vi "00_FRA_sensors_main.vi"() -> ()   [LabVIEW 2013]
uses:
  subVIs/Sensor_power_ctrl.ctl
  subVIs/Unit_select_s_m.ctl
  subVIs/UDP_read_datagram.ctl
  subVIs/UI_states.ctl
  subVIs/Global Status bar event.vi
  subVIs/loop error, restart vi_err_cluster.vi
  subVIs/loop error, restart vi.vi
  <vilib>/Utility/file.llb/Read From Spreadsheet File (string).vi
panel:
  out "Status Bar VI":string
  out "Status":string="Ready!"
  in  "Tab Control":enum32{"Settings", "Measurement", "Log", "."}(tab)
  in  "Unit select single/mult 2":T1 caption="Unit selection \nsingle/multiple"
  in  "UseAMO":bool caption="Use Amonia Sensor"
  in  "MODECN":u8 format="%08b"
  in  "REFCN":u8 format="%08b"
  in  "TIACN":u8=18 format="%05b"
  in  "Conf.set":u8=6 caption="Configuration set (Electrochemical) (0-15)" max=15 step=1
  out "ACK'd_clients":u8[](array[numeric])
  out "Number of clients":i32
  out "Export Folder Path":path
  in  "Unit selection":u8=255
  in  "Reset Unit":bool
  in  "Trigger ON":bool
  in  "Trigger OFF":bool
  in  "Period (s)":sgl=1.0 min=0.1 max=25 step=0.1
  in  "Unit selection multiple":string[][](table)
  out "Unit display A":dbl[][](graph)=[[528.1875, 527.4375, 528.1875, 527.25, 525.75, 520.125, 579.0, 800.8125, 526.6875, 524.25, 525.0, 525.1875]]
  in  "unit to show A":u8=13
  out "Unit display B":dbl[][](graph)=[[543.375, 541.5, 544.875, 5008.6875, 535.6875, 535.3125, 535.875, 537.5625, 538.3125, 0.5625, 571.6875, 538.3125]]
  in  "unit to show C":u8=11
  in  "unit to show D":u8=12
  out "Unit display D":dbl[][](graph)=[[-0.01530459835686071, -0.000554118739038989, 0.03629888532152492, 0.0025318779311733763, 0.030571059615454033, 0.00759975996654827, 0.0011509882323559317, 0.003101779382480796, 0.003088657192881872, -0.0032983569178113292, -0.0038528679526479426, 1.0]]
  out "Unit display C":dbl[][](graph)=[[-0.01530459835686071, -0.000554118739038989, 0.03629888532152492, 0.0025318779311733763, 0.030571059615454033, 0.00759975996654827, 0.0011509882323559317, 0.003101779382480796, 0.003088657192881872, -0.0032983569178113292, -0.0038528679526479426, 1.0]]
  in  "unit to show B":u8=14
  out "Dead Units":u8[](array[numeric])
  out "Logged status messages":string[][](table)
  out "Unit selection merged":u8[][](array[numeric])
  in  "update_legends":bool
  out "Alive Units":u8[](array[numeric])
  out "Answer_received_from":u8[](array[numeric])
  in  "Unit port":u16=65500
  out "Data file ref":refnum<file>
  in  "Sensor power control":T2={"Power A1.0"=TRUE, "Power A1.1"=TRUE, "Power A1.2"=TRUE, "Power A1.3"=TRUE, "Power A2.0"=TRUE, "Power A2.1"=TRUE, "Power A2.2"=TRUE, "Power A2.3"=TRUE, "Power A3.1"=TRUE, "Power A3.2"=TRUE}
  in  "Power all sensors ON/OFF":bool
  out "ACK'd_clients addr":u32[](array[numeric]) format="%x"
  out "address":u32 format="%08x"
  out "data received":string
  out "Datagram to send":string
  in  "Stop Button":bool
  # "Single or all units configuration"
  # "Multiple units / custom"
  # "Port A3.1 is overritten by custom values in some sets"
  # "default 14k gain"
  # "Enter 255 (broadcast) for all units (also not ACK'd)"
  # "default 20%VDD"
  # "Period setting will be ignored - 250ms will be used\nTGS2444 must be in A3.2 port\nPriority over El-Chem sensors"
  # "default 0  - means turned off"
  # "LMP91000 analog front end configuration\n0 - no electrochemical sensors will be configured\n1-15 - Electrochemical sensing with setting according to table in System spec"
  # "Apply actions panel"
  # "Stop will stop LabVIEW logging\nregardless of unit selection"
  # "ACK sent to units from VI start"
  # "Sends to all ACK'd"
  # "variables and settings"
  # "Manual override for power"
  # "Do not use!\nAll sensors are powered\npermanenty.\n\nSome require power patten,\nso Unit switches them as needed"
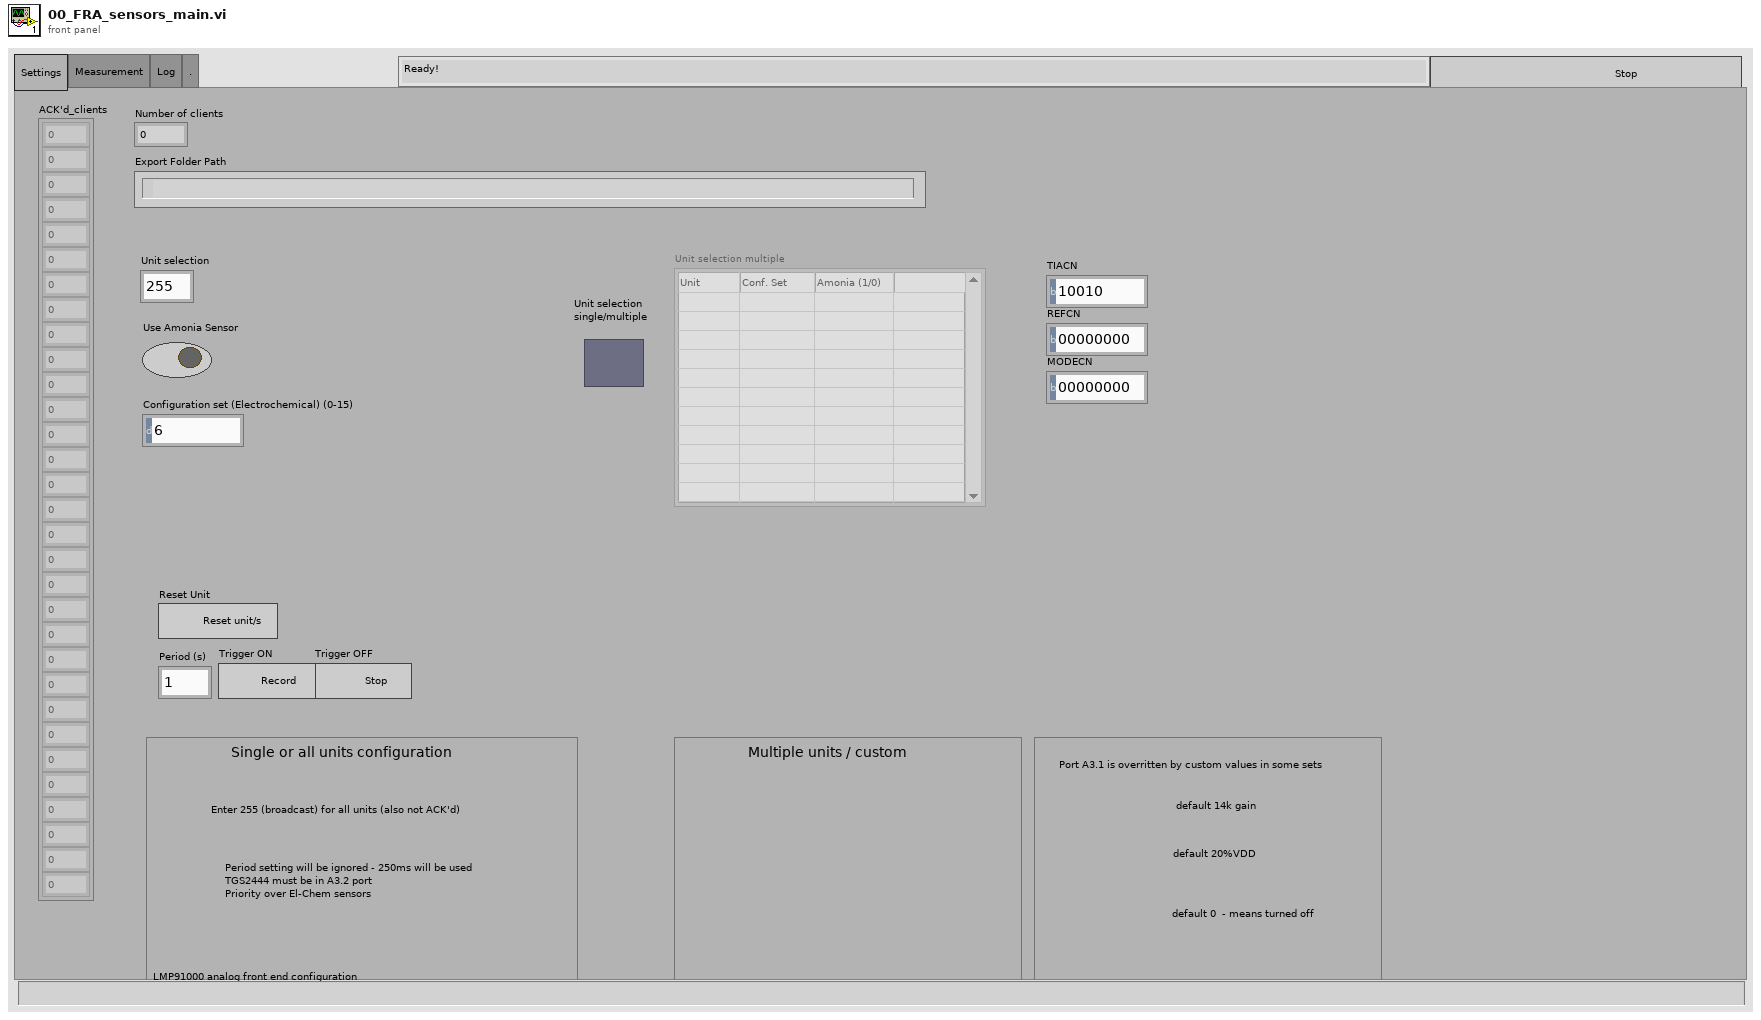
[diagram p1: front panel]
types:
  T1 = typedef "Unit_select_s_m.ctl" = bool
  T2 = typedef "Sensor_power_ctrl.ctl" = cluster{"Power A1.0":bool, "Power A1.1":bool, "Power A1.2":bool, "Power A1.3":bool, "Power A2.0":bool, "Power A2.1":bool, "Power A2.2":bool, "Power A2.3":bool, "Power A3.1":bool, "Power A3.2":bool}
  T3 = enum16{"open", "replace", "create", "open or create", "replace or create", "replace or create with confirmation"}
  T4 = typedef "UI_states.ctl" = enum16{"SENS_PWR_ALL_ON_OFF", "INIT", "IDLE", "RUN", "STOP", "SENS_PWR_CTRL", "UNIT_RESET", "MEAS_TRIG_ON", "MEAS_TRIG_OFF", "UPD_LEG", ""}
  T5 = typedef "UDP_read_datagram.ctl" = cluster{"msg":string, "address":u32, "port":u16}
  T6 = enum8{"Enabled", "Disabled", "Disabled and Grayed Out"}
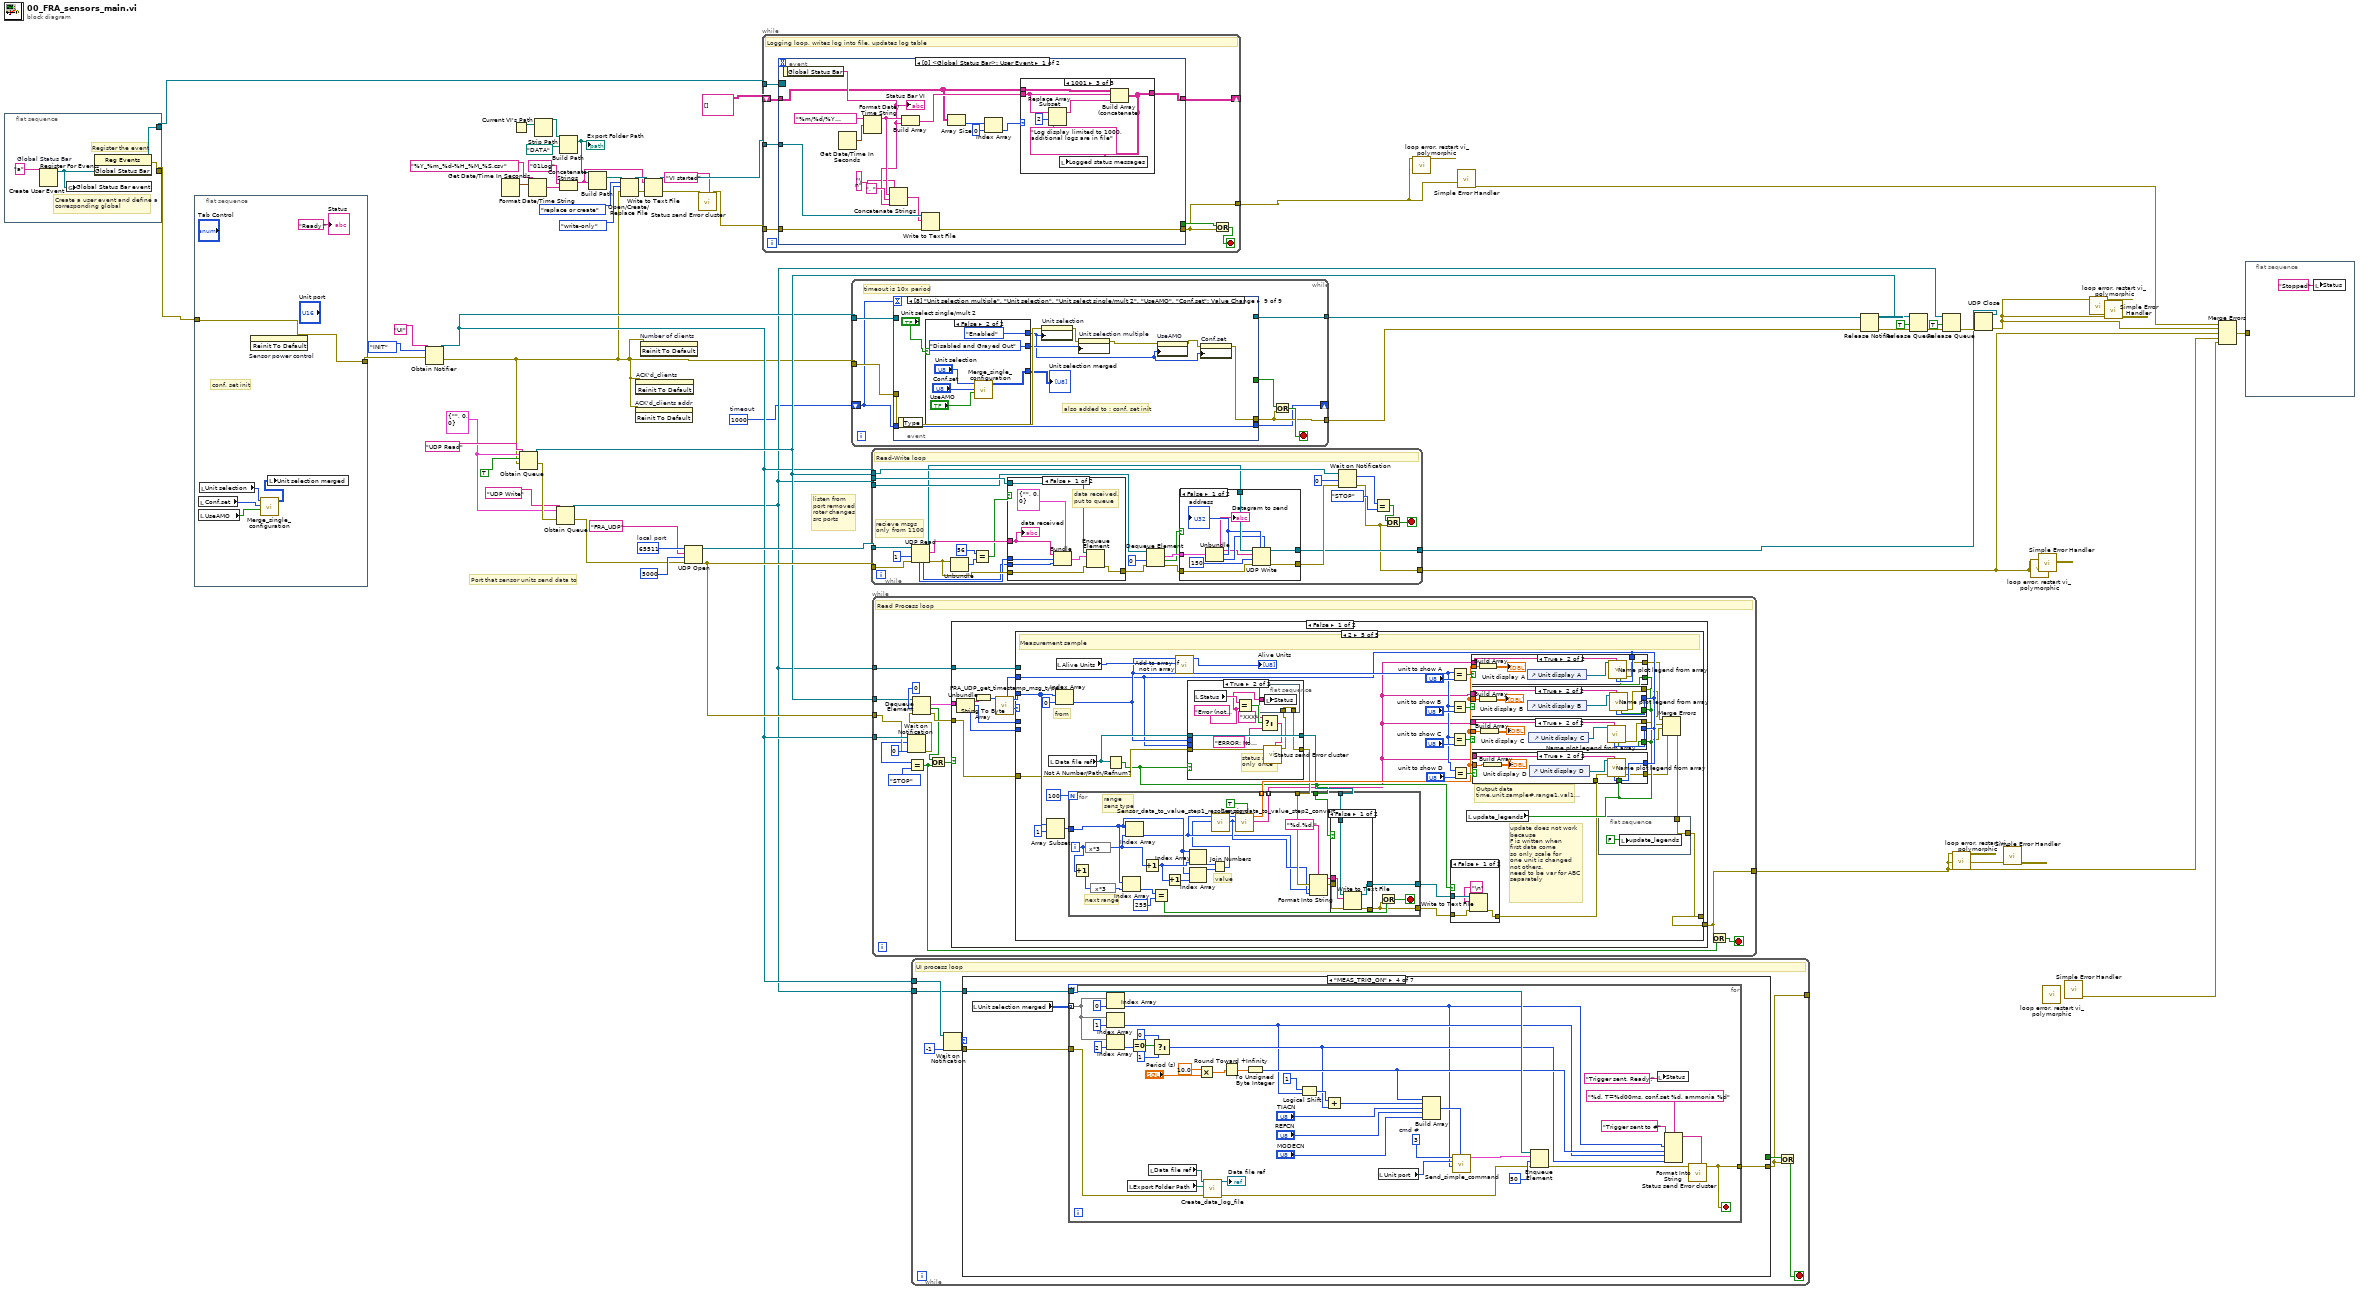
[diagram p0: block diagram]
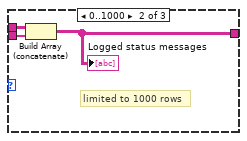
[diagram p3: hidden frame]
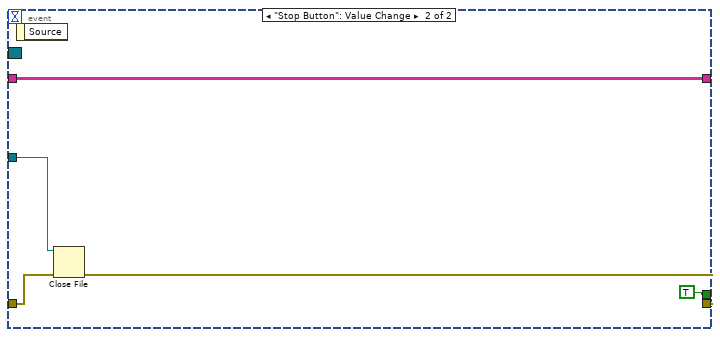
[diagram p4: hidden frame]
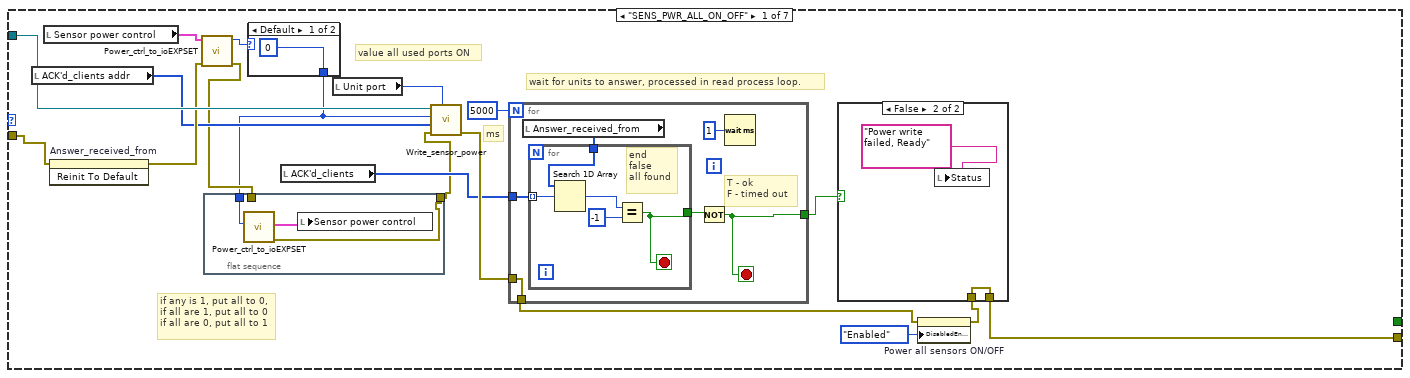
[diagram p5: hidden frame]
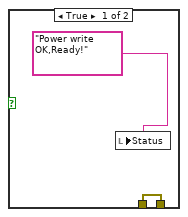
[diagram p6: hidden frame]
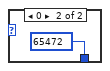
[diagram p7: hidden frame]
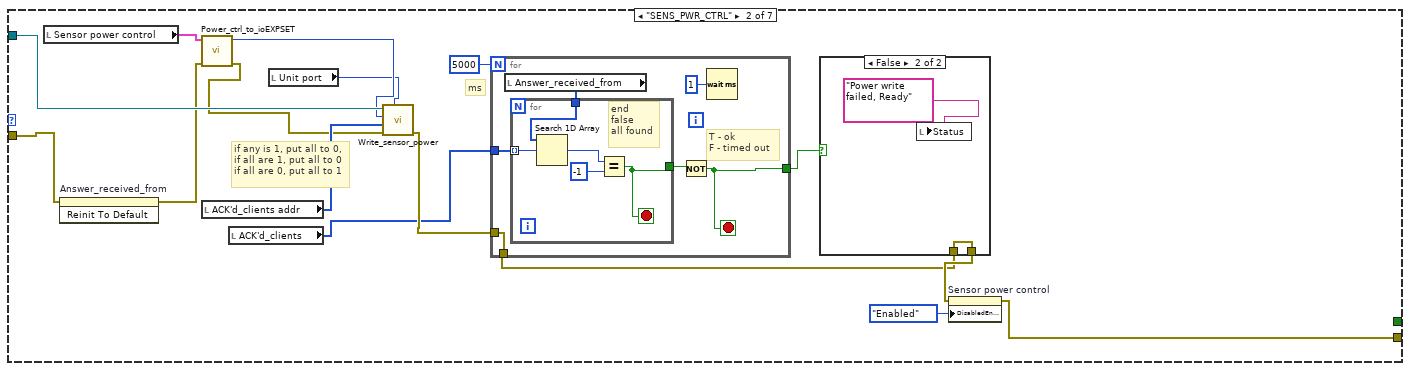
[diagram p8: hidden frame]
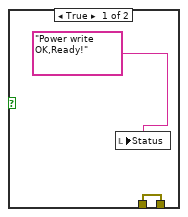
[diagram p9: hidden frame]
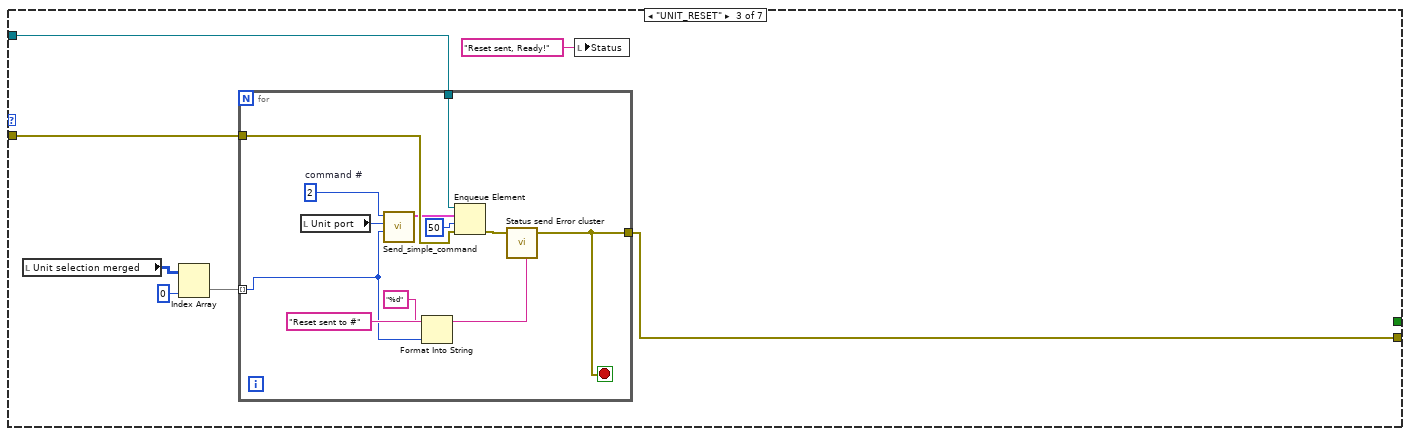
[diagram p10: hidden frame]
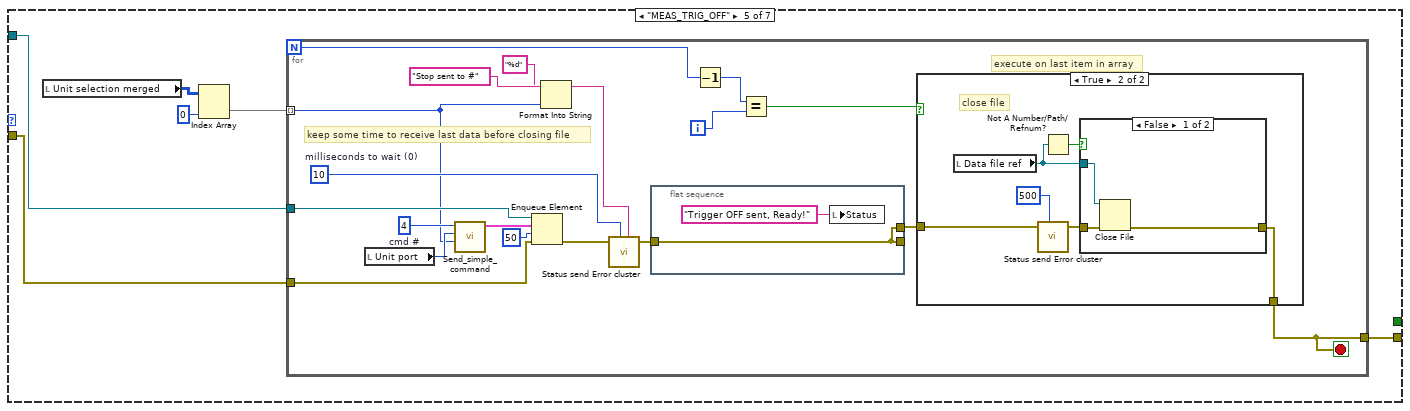
[diagram p11: hidden frame]
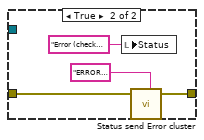
[diagram p13: hidden frame]
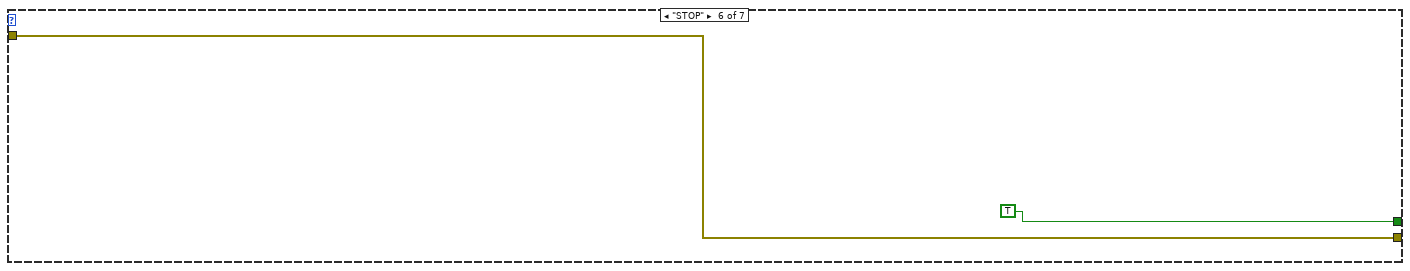
[diagram p14: hidden frame]
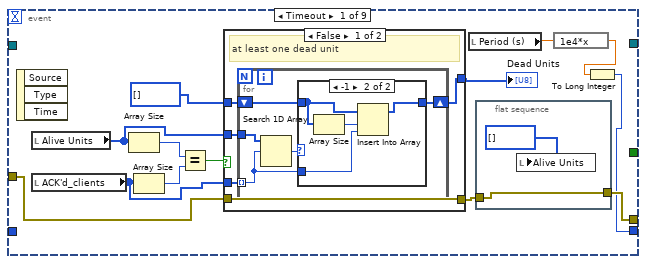
[diagram p16: hidden frame]
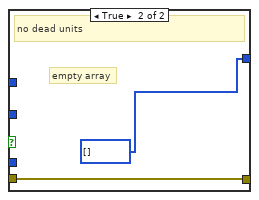
[diagram p18: hidden frame]
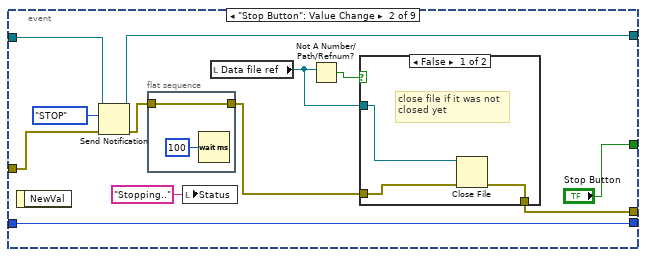
[diagram p19: hidden frame]
diagram:
  w1 = 1000  # timeout
  w37 = T5 {"msg"="", "address"=0, "port"=0}
  w55 = u16 65511  # local port
  # "listen from\nport removed\nroter changes\nsrc ports"
  # "Port that sensor units send data to"
  n1 = flat-sequence {
    tunnel: [w57] -> w14
    tunnel: [w56] -> w13
    frame #0 {
      w58 = "a"  # Global Status Bar
      # "Register the event"
      # "Create a user event and define a corresponding global"
      n2 = Create User Event(user event datatype=w58) -> (user event=w59:refnum<user-event>)  [unwired: 1 in, 1 out]
      n3 = global write "Global Status bar event.vi" "Global Status Bar event"(w59) -> ()
      n4 = register-events(w59) -> (reference out=w56:refnum<event-registration>, error out=w57:errorcluster)  [unwired: 2 in]
    }
  }
  n5 = flat-sequence {
    tunnel: [w64] -> w48
    tunnel: w14 -> [w64]
    frame #0 {
      # "conf. set init"
      n6 = local read "Conf.set"() -> (w62:u8)
      n7 = local read "UseAMO"() -> (w61:bool)
      n8 = local read "Unit selection"() -> (w63:u8)
      n9 = invoke on="Sensor power control" class="Clust (strict)" method="Reinit To Default"() -> ()  [unwired: 3 in, 3 out]
      n10 = call "Merge_single_configuration.vi"("UseAMO"=w61, "Conf.set"=w62, "Unit selection"=w63) -> ("Array"=w60:u8[][])  [unwired: 8 in]
      n11 = local write "Unit selection merged"(w60) -> ()
      "Status" <- "Ready!" ("Status")
    }
  }
  n12 = Obtain Notifier(name (unnamed)="UI", notification data type=UI_states."INIT" ("Enum"), error in (no error)=w48) -> (notifier out=w31:refnum<notifier>, error out=w16:errorcluster)  [unwired: 1 in, 1 out]
  n13 = Get Date/Time In Seconds() -> (seconds since 1Jan1904=w29:timestamp)
  n14 = Current VI's Path() -> (path=w25:path)
  n15 = Obtain Queue(name (unnamed)="UDP Read", element data type=w37, create if not found? (T)=TRUE, error in (no error)=w16) -> (queue out=w34:refnum<queue>, error out=w39:errorcluster)  [unwired: 1 in, 1 out]
  n16 = Format Date/Time String(time format string (%c)="%Y_%m_%d-%H_%M_%S.csv", seconds (now)=w29) -> (date/time string=w17:string)  [unwired: 1 in]
  n17 = Strip Path(path=w25) -> (stripped path=w26:path)  [unwired: 1 out]
  n18 = Obtain Queue(name (unnamed)="UDP Write", element data type=w37, error in (no error)=w39) -> (queue out=w30:refnum<queue>, error out=w36:errorcluster)  [unwired: 2 in, 1 out]
  n19 = Build Path(base path=w26, name or relative path=path "DATA") -> (appended path=w6:path)
  "Export Folder Path" <- w6
  n20 = Concatenate Strings("01Log" ("name or relative path"), w17) -> (w18:string)
  n21 = Build Path(base path=w6, name or relative path=w18) -> (appended path=w24:path)
  n22 = Open/Create/Replace File(file path (use dialog)=w24, error in=w16, operation (0:open)=T3."replace or create", access (0:read/write)=enum16{"read/write", "read-only", "write-only"}."write-only") -> (refnum out=w21:refnum<file>, error out=w20:errorcluster)  [unwired: 2 in, 1 out]
  n23 = invoke on="ACK'd_clients addr" class="Arr (strict)" method="Reinit To Default"(error in=w16) -> ()  [unwired: 2 in, 3 out]
  n24 = invoke on="ACK'd_clients" class="Arr (strict)" method="Reinit To Default"(error in=w16) -> ()  [unwired: 2 in, 3 out]
  n25 = invoke on="Number of clients" class="DigNum (strict)" method="Reinit To Default"(error in=w16) -> ()  [unwired: 2 in, 3 out]
  n26 = Write to Text File(file (use dialog)=w21, text=w18, error in=w20) -> (refnum out=w12:refnum<file>, error out=w11:errorcluster)  [unwired: 1 in, 1 out]
  n27 = UDP Open(8:w36, 9:5000 ("timeout ms (25000)"), 10:"FRA_UDP" ("service name"), 11:w55) -> (port=w49:refnum<k16>, 0:w50:errorcluster)  [unwired: 1 in, 1 out]
  n28 = call "Status send Error cluster.vi"("error in (no error)"=w11, "Send status msg \"XXX\" or don't wire for no message"="VI started" ("Send status msg \"XXX\" or don't wire for no message")) -> ("error out"=w10:errorcluster)  [unwired: 7 in]
  n29 = while {
    shift-right: [w71] -> _
    shift-left: string[][] [] -> [w72]
    tunnel: w13 -> [w73]
    tunnel: w12 -> [w68]
    tunnel: [w67] -> w5
    tunnel: w10 -> [w66]
    stop <- w70 stop-if-true
    # "Logging loop, writes log into file, updates log table"
    n30 = event shown="[0] <Global Status Bar>: User Event" {
      selector: w73 -> [_ _]
      dyn-events: _ -> [_ _]
      timeout: _ -> [_ _]
      tunnel: w72 -> [w77 w103]
      tunnel: [w86 w103] -> w71
      tunnel: [w79 w101] -> w67
      tunnel: [_ TRUE] -> w69
      tunnel: w68 -> [w85 w102]
      tunnel: w66 -> [w78 w100]
      event User Event {
        n31 = event-data() -> ("Global Status Bar"=w82:string)  [unwired: 1 in]
        "Status Bar VI" <- w82
        n32 = Get Date/Time In Seconds() -> (seconds since 1Jan1904=w88:timestamp)
        n33 = Format Date/Time String(time format string (%c)="%m/%d/%Y    %H:%M:%S%3u", seconds (now)=w88) -> (date/time string=w84:string)  [unwired: 1 in]
        n34 = Concatenate Strings("\n" ("text"), w84, ", " ("string"), w82) -> (w80:string)
        n35 = Build Array(w84, w82) -> (w89:string[])
        n36 = Write to Text File(file (use dialog)=w85, text=w80, error in=w78) -> (error out=w79:errorcluster)  [unwired: 1 in, 2 out]
        n37 = Array Size(array=w77) -> (size(s)=w76:i32[])
        n38 = Index Array(array=w76, index=0) -> (element=w74:i32)
        n39 = case shown="1001" w74 {
          tunnel: w89 -> [_ w93 w98]
          tunnel: w77 -> [w90 w92 w99]
          tunnel: [w90 w91 w94] -> w86
          frame Default {
          }
          frame 0..1000 {
            # "limited to 1000 rows"
            n40 = Build Array (concatenate)(w92, w93) -> (w91:string[][])
            "Logged status messages" <- w91
          }
          frame 1001 {
            n41 = Replace Array Subset(array=w98, new element="Log display limited to 1000, additional logs are in file" ("new element/subarray"), index=2) -> (w95:string[])
            n42 = Build Array (concatenate)(w99, w98, w95) -> (w94:string[][])
            n43 = local write "Logged status messages"(w94) -> ()
          }
        }
      }
      event "Stop Button": Value Change {
        n44 = event-data() -> ()  [unwired: 1 in, 1 out]
        n45 = Close File(refnum=w102, error in=w100) -> (error out=w101:errorcluster)  [unwired: 1 out]
      }
    }
    n46 = Or(x=w69, y=w67) -> (x .or. y?=w70:bool)
  }
  n47 = while {
    tunnel: w31 -> [w112]
    tunnel: w16 -> [w111]
    tunnel: [w108] -> w45
    tunnel: [w107] -> w44
    shift-right: [w105] -> _
    shift-left: w1 -> [w106]
    stop <- w109 stop-if-true
    # "timeout is 10x period"
    n48 = event shown="[8] \"Unit selection multiple\", \"Unit selection\", \"Unit select single/mult 2\", \"UseAMO\", \"Conf.set\": Value Change" {
      selector: _ -> [_ _ _ _ _ _ _ _ _]
      dyn-events: _ -> [_ _ _ _ _ _ _ _ _]
      timeout: w106 -> [_ _ _ _ _ _ _ _ _]
      tunnel: w112 -> [_ w155 w170 w188 w202 w209 w215 _ _]
      tunnel: [w116 w146 w167 w186 w200 w210 w216 w220 w223] -> w107
      tunnel: w111 -> [w122 w153 w168 w185 w203 _ w217 w220 w230]
      tunnel: [_ "Stop Button" _ _ _ _ _ _ _] -> w110
      tunnel: [_ w152 w169 w187 w201 w208 w214 _ _] -> w108
      tunnel: w106 -> [_ w149 w163 w181 w199 w206 w212 w218 w228]
      tunnel: [w113 w149 w163 w181 w199 w206 w212 w218 w228] -> w105
      event Timeout {
        n49 = event-data() -> ()  [unwired: 1 in, 3 out]
        n50 = local read "Alive Units"() -> (w120:u8[])
        n51 = local read "ACK'd_clients"() -> (w121:u8[])
        n52 = Array Size(array=w120) -> (size(s)=w125:i32)
        n53 = Array Size(array=w121) -> (size(s)=w124:i32)
        n54 = Equal?(x=w125, y=w124) -> (x = y?=w123:bool)
        n55 = case shown="False" w123 {
          tunnel: w122 -> [w128 w144]
          tunnel: [w128 w144] -> w117
          tunnel: w121 -> [w132 _]
          tunnel: w120 -> [w131 _]
          tunnel: u8[] [] ("Alive Units") -> [w130 _]
          tunnel: [w129 u8[] [] ("Alive Units")] -> w118
          frame False {
            # "at least one dead unit"
            n56 = for {
              tunnel: w132 -> [w135] mode=indexing
              tunnel: w131 -> [w137]
              shift-right: [w133] -> w129
              shift-left: w130 -> [w134]
              n57 = Search 1D Array(1D array=w137, element=w135) -> (index of element=w136:i32)  [unwired: 1 in]
              n58 = case shown="-1" w136 {
                tunnel: w135 -> [_ w142]
                tunnel: w134 -> [w138 w140]
                tunnel: [w138 w139] -> w133
                frame Default {
                }
                frame -1 {
                  n59 = Array Size(array=w140) -> (size(s)=w141:i32)
                  n60 = Insert Into Array(array=w140, index=w141, new element=w142) -> (w139:u8[])
                }
              }
            }
          }
          frame True {
            # "empty array"
            # "no dead units"
          }
        }
        "Dead Units" <- w118
        n61 = local read "Period (s)"() -> (w115:sgl)
        n62 = flat-sequence {
          tunnel: w117 -> [w127]
          tunnel: [w127] -> w116
          frame #0 {
            n63 = local write "Alive Units"(u8[] [] ("Alive Units")) -> ()
          }
        }
        n64 = expression code="1e4*x"(w115) -> (w114:sgl)
        n65 = To Long Integer(number=w114) -> (32bit integer=w113:i32)
      }
      event "Stop Button": Value Change {
        n66 = event-data() -> ()  [unwired: 1 in, 1 out]
        n67 = Send Notification(notification=UI_states."STOP", notifier=w155, error in (no error)=w153) -> (notifier out=w152:refnum<notifier>, error out=w151:errorcluster)
        n68 = flat-sequence {
          tunnel: w151 -> [w161]
          tunnel: [w161] -> w148
          frame #0 {
            n69 = Wait (ms)(milliseconds to wait=u32 100) -> ()  [unwired: 1 out]
          }
        }
        n70 = local write "Status"("Stopping.." ("Status")) -> ()
        n71 = local read "Data file ref"() -> (w145:refnum<file>)
        n72 = Not A Number/Path/Refnum?(number/path/refnum=w145) -> (NaN/Path/Refnum?=w147:bool)
        n73 = case shown="False" w147 {
          tunnel: w148 -> [w158 w160]
          tunnel: [w157 w160] -> w146
          tunnel: w145 -> [w159 _]
          frame False {
            # "close file if it was not\nclosed yet"
            n74 = Close File(refnum=w159, error in=w158) -> (error out=w157:errorcluster)  [unwired: 1 out]
          }
          frame True {
          }
        }
      }
      event "Power all sensors ON/OFF": Value Change {
        n75 = event-data() -> ()  [unwired: 1 in, 1 out]
        n76 = local read "ACK'd_clients"() -> (w165:u8[])
        n77 = local write "Status"("Setting power..." ("Status")) -> ()
        n78 = Array Size(array=w165) -> (size(s)=w164:i32)
        n79 = case shown="Default" w164 {
          tunnel: w170 -> [w173 w179]
          tunnel: [w173 w178] -> w169
          tunnel: w168 -> [w172 w176]
          tunnel: [w172 w174] -> w167
          frame 0 {
            n80 = local write "Status"("No clients, power not set!, Ready" ("Status")) -> ()
          }
          frame Default {
            n81 = property on="Power all sensors ON/OFF" class="Bool"(error in=w176, "DisabledEnum"=T6."Disabled and Grayed Out" ("Disabled")) -> (error out=w175:errorcluster)  [unwired: 1 in, 1 out]
            n82 = Send Notification(notification=UI_states."SENS_PWR_ALL_ON_OFF", notifier=w179, error in (no error)=w175) -> (notifier out=w178:refnum<notifier>, error out=w174:errorcluster)
          }
        }
      }
      event Value Change {
        n83 = event-data() -> ()  [unwired: 1 in, 1 out]
        n84 = local read "ACK'd_clients"() -> (w183:u8[])
        n85 = local write "Status"("Setting power..." ("Status")) -> ()
        n86 = Array Size(array=w183) -> (size(s)=w182:i32)
        n87 = case shown="0" w182 {
          tunnel: w188 -> [w190 w197]
          tunnel: [w190 w196] -> w187
          tunnel: [w191 w195] -> w186
          tunnel: w185 -> [w191 w193]
          frame 0 {
            n88 = local write "Status"("No clients, power not set!, Ready" ("Status")) -> ()
          }
          frame Default {
            n89 = property on="Sensor power control" class="Clust (strict)"(error in=w193, "DisabledEnum"=T6."Disabled and Grayed Out" ("Disabled")) -> (error out=w194:errorcluster)  [unwired: 1 in, 1 out]
            n90 = Send Notification(notification=UI_states."SENS_PWR_CTRL", notifier=w197, error in (no error)=w194) -> (notifier out=w196:refnum<notifier>, error out=w195:errorcluster)
          }
        }
      }
      event "Reset Unit": Value Change {
        n91 = event-data() -> ()  [unwired: 1 in, 1 out]
        n92 = local write "Status"("Resetting unit/s..." ("Status")) -> ()
        n93 = Send Notification(notification=UI_states."UNIT_RESET", notifier=w202, error in (no error)=w203) -> (notifier out=w201:refnum<notifier>, error out=w200:errorcluster)
      }
      event "Trigger ON": Value Change {
        n94 = event-data() -> ()  [unwired: 1 in, 1 out]
        n95 = Send Notification(notification=UI_states."MEAS_TRIG_ON", notifier=w209) -> (notifier out=w208:refnum<notifier>, error out=w210:errorcluster)  [unwired: 1 in]
      }
      event "Trigger OFF": Value Change {
        n96 = event-data() -> ()  [unwired: 1 in, 1 out]
        n97 = Send Notification(notification=UI_states."MEAS_TRIG_OFF", notifier=w215, error in (no error)=w217) -> (notifier out=w214:refnum<notifier>, error out=w216:errorcluster)
        n98 = local write "Status"("Stopping measurement..." ("Status")) -> ()
      }
      event "unit to show A", "unit to show B", "unit to show C", "unit to show D", "update_legends": Value Change {
        # "when you change unit display while running\nlegend update should be invoked"
        n99 = event-data() -> ()  [unwired: 1 in, 2 out]
        n100 = local write "update_legends"(TRUE ("update_legends")) -> ()
      }
      event "Unit selection multiple", "Unit selection", "UseAMO", "Conf.set": Value Change {
        # "also added to : conf. set init"
        n101 = event-data() -> ()  [unwired: 1 in, 1 out]
        n102 = case shown="False" "Unit select single/mult 2" {
          tunnel: [T6."Disabled and Grayed Out" ("Disabled") T6."Enabled" ("Disabled")] -> w221
          tunnel: [T6."Enabled" ("Disabled") T6."Disabled and Grayed Out" ("Disabled")] -> w227
          tunnel: [w231 w237] -> w226
          frame True {
            n103 = Decimal String To Number(string="Unit selection multiple") -> (number=w233:i32[][])  [unwired: 2 in, 1 out]
            n104 = To Unsigned Byte Integer(number=w233) -> (unsigned 8bit integer=w231:u8[][])
          }
          frame False {
            n105 = call "Merge_single_configuration.vi"("UseAMO"="UseAMO", "Conf.set"="Conf.set", "Unit selection"="Unit selection") -> ("Array"=w237:u8[][])  [unwired: 8 in]
          }
        }
        "Unit selection merged" <- w226
        n106 = property on="Unit selection" class="DigNum (strict)"(error in=w230, "DisabledEnum"=w221) -> (error out=w229:errorcluster)  [unwired: 1 in, 1 out]
        n107 = property on="Unit selection multiple" class="Tbl (strict)"(error in=w229, "DisabledEnum"=w227) -> (error out=w222:errorcluster)  [unwired: 1 in, 1 out]
        n108 = property on="UseAMO" class="Bool (strict)"(error in=w222, "DisabledEnum"=w221) -> (error out=w224:errorcluster)  [unwired: 1 in, 1 out]
        n109 = property on="Conf.set" class="DigNum (strict)"(error in=w224, "DisabledEnum"=w221) -> (error out=w223:errorcluster)  [unwired: 1 in, 1 out]
      }
    }
    n110 = Or(x=w110, y=w107) -> (x .or. y?=w109:bool)
  }
  n111 = while {
    tunnel: w34 -> [w257]
    tunnel: w50 -> [w262]
    tunnel: w49 -> [w267]
    tunnel: w31 -> [w266]
    tunnel: w30 -> [w254]
    tunnel: [w248] -> w35
    tunnel: [w245] -> w3
    stop <- w246 stop-if-true
    # "recieve msgs\nonly from 1100"
    # "Read-Write loop"
    n112 = UDP Read(connection ID=w267, timeout ms (25000)=1, 8:w262) -> (data out=w258:string, error out=w259:errorcluster, 3:w252:refnum<k16>, 4:w244:u16, 6:w256:u32)  [unwired: 1 out]
    n113 = Unbundle(w259) -> ("code"=w261:i32)  [unwired: 2 out]
    n114 = Equal?(x=56, y=w261) -> (x = y?=w243:bool)
    n115 = case shown="False" w243 {
      tunnel: w259 -> [w287 _]
      tunnel: [w282 errorcluster {"status"=FALSE, "code"=0, "source"=""} ("error out")] -> w251
      tunnel: w258 -> [w280 _]
      tunnel: w257 -> [w281 _]
      tunnel: w256 -> [w284 _]
      tunnel: w244 -> [w283 _]
      frame False {
        # "data received, \nput to queue"
        n116 = Bundle(cluster=T5 {"msg"="", "address"=0, "port"=0}, "msg"=w280, "address"=w284, "port"=w283) -> (w286:T5)
        n117 = Enqueue Element(queue=w281, element=w286, error in (no error)=w287) -> (error out=w282:errorcluster)  [unwired: 1 in, 2 out]
        "data received" <- w280
      }
      frame True {
        # "timeout heppened\nno data received"
      }
    }
    n118 = Dequeue Element(queue=w254, timeout in ms (-1)=0, error in (no error)=w251) -> (element=w253:T5, timed out?=w249:bool, error out=w242:errorcluster)  [unwired: 1 out]
    n119 = case shown="False" w249 {
      tunnel: w253 -> [w277 _]
      tunnel: w252 -> [w276 w278]
      tunnel: w242 -> [w274 w279]
      tunnel: [w271 w279] -> w250
      tunnel: [w270 w278] -> w248
      frame False {
        n120 = Unbundle(w277) -> ("msg"=w269:string, "address"=w273:u32, "port"=w272:u16)
        "Datagram to send" <- w269
        "address" <- w273
        n121 = UDP Write(address=w273, port or service name=w272, connection ID=w276, data in=w269, 8:w274, 9:150 ("timeout ms (25000)")) -> (error out=w271:errorcluster, 3:w270:refnum<k16>)
      }
      frame True {
        # "no message in send buffer"
      }
    }
    n122 = Wait on Notification(notifier=w266, timeout in ms (-1)=0, error in (no error)=w250) -> (notification=w264:T4, error out=w245:errorcluster)  [unwired: 1 in, 2 out]
    n123 = Equal?(x=w264, y=UI_states."STOP") -> (x = y?=w247:bool)
    n124 = Or(x=w247, y=w245) -> (x .or. y?=w246:bool)
  }
  n125 = while {
    tunnel: w50 -> [w296]
    tunnel: w34 -> [w303]
    tunnel: w31 -> [w297]
    tunnel: w30 -> [w300]
    tunnel: [w293] -> w2
    stop <- w294 stop-if-true
    # "Read Process loop"
    n126 = Wait on Notification(notifier=w297, timeout in ms (-1)=0, error in (no error)=w296) -> (notification=w289:T4, error out=w295:errorcluster)  [unwired: 1 in, 2 out]
    n127 = Equal?(x=w289, y=UI_states."STOP") -> (x = y?=w292:bool)
    n128 = Dequeue Element(queue=w303, timeout in ms (-1)=0, error in (no error)=w295) -> (element=w301:T5, timed out?=w290:bool, error out=w302:errorcluster)  [unwired: 1 out]
    n129 = Or(x=w290, y=w292) -> (x .or. y?=w291:bool)
    n130 = case shown="False" w291 {
      tunnel: w302 -> [w306 w508]
      tunnel: w301 -> [w313 _]
      tunnel: [w305 w508] -> w293
      tunnel: w300 -> [w308 _]
      frame False {
        n131 = Unbundle(w313) -> ("msg"=w312:string, "address"=w309:u32, "port"=w307:u16)
        n132 = String To Byte Array(string=w312) -> (unsigned byte array=w315:u8[])
        n133 = call "FRA_UDP_get_timestamp_msg_type.vi"("incoming_UDP"=w315) -> ("MSG_type_byte"=w314:u8, "datagram_rest"=w311:u8[], "Datagram number"=w310:u32)  [unwired: 6 in, 2 out]
        n134 = case shown="2" w314 {
          tunnel: w311 -> [_ _ w345 w361 w417]
          tunnel: w310 -> [_ _ _ _ w393]
          tunnel: w309 -> [_ w320 _ _ _]
          tunnel: w308 -> [_ w330 _ _ _]
          tunnel: w307 -> [_ w332 _ _ _]
          tunnel: w306 -> [w316 w328 w340 w365 w402]
          tunnel: [w316 w325 w341 w357 w385] -> w305
          frame 0, Default {
          }
          frame 4 {
            # "add client to list if not there already"
            # "sensor unit annoucement"
            n135 = call "FRA_UDP_send_ACK.vi"() -> ("Datagram to send"=w333:string)  [unwired: 11 in]
            n136 = local read "ACK'd_clients addr"() -> (w327:u32[])
            n137 = Bundle(cluster=T5 {"msg"="", "address"=0, "port"=0}, "msg"=w333, "address"=w320, "port"=w332) -> (w331:T5)
            n138 = Enqueue Element(queue=w330, element=w331, timeout in ms (-1)=100, error in (no error)=w328) -> (error out=w326:errorcluster)  [unwired: 2 out]
            n139 = call "Add to array if not in array.vi"("Array in"=w327, "Number to add"=w320) -> ("New array size"=→"Number of clients":i32, "Array out"=w318:u32[])  [unwired: 8 in]
            "ACK'd_clients addr" <- w318
            n140 = To Unsigned Byte Integer(number=w320) -> (unsigned 8bit integer=w321:u8)
            n141 = Format Into String(format string="%d", initial string="Announcement from #", w321) -> (resulting string=w324:string)  [unwired: 1 in, 1 out]
            n142 = call "Status send Error cluster.vi"("error in (no error)"=w326, "Send status msg \"XXX\" or don't wire for no message"=w324) -> ("error out"=w325:errorcluster)  [unwired: 7 in]
            n143 = To Unsigned Byte Integer(number=w318) -> (unsigned 8bit integer=→"ACK'd_clients":u8[])
          }
          frame 3 {
            # "sender identification"
            # "error code, byte 6"
            # "@TODO\nadd to file save"
            # "row is an error code"
            # "Error report from unit"
            n144 = Current VI's Path() -> (path=w348:path)
            n145 = Index Array(array=w345, index=1) -> (element=w350:u8)
            n146 = Index Array(array=w345, index=0) -> (element=w339:u8)
            n147 = Strip Path(path=w348) -> (stripped path=w347:path)  [unwired: 1 out]
            n148 = Build Path(base path=w347, name or relative path="error_codes.csv") -> (appended path=w355:path)
            n149 = call-poly <vilib>:"Read From Spreadsheet File.vi"("delimiter (\\t)"="," ("delimiter (\\t)"), "file path (dialog if empty)"=w355) -> ("all rows"=w352:string[][])  [unwired: 5 in, 4 out]
            n150 = To Long Integer(number=w350) -> (32bit integer=w349:i32)
            n151 = local write "Status"("Error (check log), Ready!" ("Status")) -> ()
            n152 = Index Array(array=w352, index (row)=w349, index (col)=1 ("disabled index (col)")) -> (element=w336:string)
            n153 = To Unsigned Byte Integer(number=w339) -> (unsigned 8bit integer=w342:u8)
            n154 = Format Into String(format string="%d : ", initial string="ERROR from #", w342) -> (resulting string=w337:string)  [unwired: 1 in, 1 out]
            n155 = Concatenate Strings(w337, w336) -> (w338:string)
            n156 = call "Status send Error cluster.vi"("error in (no error)"=w340, "Send status msg \"XXX\" or don't wire for no message"=w338) -> ("error out"=w341:errorcluster)  [unwired: 7 in]
          }
          frame 5 {
            # "5D38 C4BB 0500 00"
            # "Power report"
            n157 = local read "Sensor power control"() -> (w366:T2)
            n158 = Index Array(array=w361, index=2) -> (element=w367:u8)
            n159 = Index Array(array=w361, index=1) -> (element=w368:u8)
            n160 = Index Array(array=w361, index=0) -> (element=w360:u8)
            n161 = Join Numbers(hi=w368, lo=w367) -> ((hi.lo)=w359:u16)
            n162 = call "Power_ctrl_to_ioEXPSET.vi"("error in (no error)"=w365, "Sensor power control"=w366) -> ("error out"=w358:errorcluster, "IO expaneder setting out"=w364:u16)  [unwired: 7 in, 1 out]
            n163 = Equal?(x=w359, y=w364) -> (x = y?=w363:bool)
            n164 = case shown="True" w363 {
              tunnel: w360 -> [w373 w381]
              tunnel: w358 -> [w374 w380]
              tunnel: [w375 w380] -> w357
              frame False {
                n165 = Format Into String(format string="%d : ", initial string="ERROR from #", w373) -> (resulting string=w376:string)  [unwired: 1 in, 1 out]
                n166 = local write "Status"("Error (check log), Ready!" ("Status")) -> ()
                n167 = Concatenate Strings(w376, "Power set is not matching!" ("error message")) -> (w371:string)
                n168 = call "Status send Error cluster.vi"("error in (no error)"=w374, "Send status msg \"XXX\" or don't wire for no message"=w371) -> ("error out"=w375:errorcluster)  [unwired: 7 in]
              }
              frame True {
                # "matching value received from"
                n169 = local read "Answer_received_from"() -> (w382:u8[])
                n170 = Array Size(array=w382) -> (size(s)=w383:i32)
                n171 = Insert Into Array(array=w382, index=w383, new element=w381) -> (→"Answer_received_from":u8[])
              }
            }
          }
          frame 2 {
            # "update does not work\nbecause\nF is written when\nfirst data come\nso only scale for \none unit is changed\nnot others.\nneed to be var for ABC \nseparately"
            # "Output data\ntime,unit,sample#,range1,val1..."
            # "from"
            # "Measurement sample"
            n172 = Array Subset(array=w417, index=1) -> (w415:u8[])  [unwired: 1 in]
            n173 = local read "Data file ref"() -> (w399:refnum<file>)
            n174 = Index Array(array=w417, index=0) -> (element=w395:u8)
            n175 = local read "Alive Units"() -> (w397:u8[])
            n176 = Not A Number/Path/Refnum?(number/path/refnum=w399) -> (NaN/Path/Refnum?=w398:bool)
            n177 = call "Add to array if not in array.vi"("Array in"=w397, "Number to add"=w395) -> ("Array out"=→"Alive Units":u32[])  [unwired: 8 in, 1 out]
            n178 = case shown="True" w398 {
              tunnel: [w431 w441] -> w404
              tunnel: w399 -> [w430 w441]
              tunnel: [w429 w432] -> w403
              tunnel: w395 -> [w428 _]
              tunnel: w402 -> [w427 w440]
              tunnel: w393 -> [w426 _]
              frame False {
                n179 = call "Write_data_to_file_time_sender_dtgn.vi"("error in (no error)"=w427, "Datagram number"=w426, "Sender number"=w428, "Byte Stream File in"=w430) -> ("error out"=w429:errorcluster, "Byte Stream File out"=w431:refnum<file>)  [unwired: 6 in]
              }
              frame True {
                w434 = "Error (not logging to file), Ready!" ("Status")
                # "status send\nonly once"
                n180 = local read "Status"() -> (w439:string)
                n181 = Equal?(x=w439, y=w434) -> (x = y?=w438:bool)
                n182 = flat-sequence {
                  tunnel: w434 -> [w443]
                  tunnel: w433 -> [w442]
                  tunnel: [w442] -> w432
                  frame #0 {
                    n183 = local write "Status"(w443) -> ()
                  }
                }
                n184 = Select(t="XXX", s=w438, f="ERROR: Not logging to file, hit start trigger!" ("Status")) -> (s? t:f=w435:string)
                n185 = call "Status send Error cluster.vi"("error in (no error)"=w440, "Send status msg \"XXX\" or don't wire for no message"=w435) -> ("error out"=w433:errorcluster)  [unwired: 7 in]
              }
            }
            n186 = for {
              N: 100 -> [_]
              tunnel: w415 -> [w493]
              tunnel: [w475] -> w405 mode=indexing
              tunnel: [w488] -> w401
              tunnel: w404 -> [w487]
              tunnel: w403 -> [w486]
              tunnel: [w482] -> w400
              tunnel: w398 -> [w481]
              tunnel: [w474] -> w394 mode=indexing
              i -> [w496]
              stop <- w489 stop-if-true
              # "next range"
              # "value"
              # "range\nsens type"
              n187 = Increment(x=w496) -> (x+1=w495:i32)
              n188 = expression code="x*3"(w496) -> (w480:i32)
              n189 = expression code="x*3"(w495) -> (w494:i32)
              n190 = Index Array(array=w493, index=w494) -> (element=w492:u8)
              n191 = Index Array(array=w493, index=w480) -> (element=w477:u8)
              n192 = Increment(x=w480) -> (x+1=w499:i32)
              n193 = Equal?(x=w492, y=u8 255) -> (x = y?=w490:bool)
              n194 = Increment(x=w499) -> (x+1=w500:i32)
              n195 = Index Array(array=w493, index=w499) -> (element=w498:u8)
              n196 = Index Array(array=w493, index=w500) -> (element=w497:u8)
              n197 = Join Numbers(hi=w498, lo=w497) -> ((hi.lo)=w476:u16)
              n198 = call "Sensor_data_to_value_step1_resolve_sign.vi"("Sensor data"=w476, "Sensor type"=w477) -> ("Sensor data resolved sign"=w478:i32, "Sensor type out"=w479:u8)  [unwired: 8 in]
              n199 = call "Sensor_data_to_value_step2_convert.vi"("Graph format (T)"=TRUE, "Sensor data resolved sign"=w478, "Sensor type"=w479) -> ("Signal legend"=w474:string, "Value ouptut"=w475:dbl)  [unwired: 7 in]
              n200 = Format Into String(format string="%d,%d,", error in=w486, w477, w478) -> (resulting string=w483:string, error out=w485:errorcluster)  [unwired: 1 in]
              n201 = case shown="False" w481 {
                tunnel: [w505 w506] -> w488
                tunnel: w487 -> [w504 w507]
                tunnel: w485 -> [w503 w506]
                tunnel: w483 -> [w502 _]
                tunnel: [w501 w507] -> w482
                frame False {
                  n202 = Write to Text File(file (use dialog)=w504, text=w502, error in=w503) -> (refnum out=w501:refnum<file>, error out=w505:errorcluster)  [unwired: 1 in, 1 out]
                }
                frame True {
                }
              }
              n203 = Or(x=w490, y=w488) -> (x .or. y?=w489:bool)
            }
            n204 = case shown="False" w398 {
              tunnel: w401 -> [w424 w425]
              tunnel: [w423 w425] -> w387
              tunnel: w400 -> [w422 _]
              frame False {
                n205 = Write to Text File(file (use dialog)=w422, text="\n", error in=w424) -> (error out=w423:errorcluster)  [unwired: 1 in, 2 out]
              }
              frame True {
              }
            }
            n206 = Equal?(x=w395, y="unit to show B") -> (x = y?=w411:bool)
            n207 = Equal?(x=w395, y="unit to show C") -> (x = y?=w408:bool)
            n208 = Equal?(x=w395, y="unit to show A") -> (x = y?=w412:bool)
            n209 = Equal?(x=w395, y="unit to show D") -> (x = y?=w407:bool)
            n210 = local read "update_legends"() -> (w392:bool)
            n211 = case shown="True" w411 {
              tunnel: w405 -> [_ w465]
              tunnel: w394 -> [_ w463]
              tunnel: w393 -> [_ w461]
              tunnel: w392 -> [_ w460]
              tunnel: [_ w459] -> w390
              frame False {
              }
              frame True {
                n212 = Build Array(w465) -> (→"Unit display B":dbl[][])
                n213 = control-ref of="Unit display B"() -> (w462:refnum<vi>)
                n214 = call "Name plot legend from array.vi"("Force write (F)"=w460, "Enabled (1-10)(1)"=w461, "Names legend"=w463, "Chart in"=w462) -> ("error out"=w459:errorcluster)  [unwired: 7 in]
              }
            }
            n215 = case shown="True" w408 {
              tunnel: w405 -> [_ w458]
              tunnel: w394 -> [_ w456]
              tunnel: w393 -> [_ w454]
              tunnel: w392 -> [_ w453]
              tunnel: [_ w452] -> w389
              frame False {
              }
              frame True {
                n216 = Build Array(w458) -> (→"Unit display C":dbl[][])
                n217 = control-ref of="Unit display C"() -> (w455:refnum<vi>)
                n218 = call "Name plot legend from array.vi"("Force write (F)"=w453, "Enabled (1-10)(1)"=w454, "Names legend"=w456, "Chart in"=w455) -> ("error out"=w452:errorcluster)  [unwired: 7 in]
              }
            }
            n219 = case shown="True" w412 {
              tunnel: w405 -> [_ w472]
              tunnel: w394 -> [_ w470]
              tunnel: w393 -> [_ w468]
              tunnel: w392 -> [_ w467]
              tunnel: [_ w466] -> w391
              frame False {
              }
              frame True {
                n220 = Build Array(w472) -> (→"Unit display A":dbl[][])
                n221 = control-ref of="Unit display A"() -> (w469:refnum<vi>)
                n222 = call "Name plot legend from array.vi"("Force write (F)"=w467, "Enabled (1-10)(1)"=w468, "Names legend"=w470, "Chart in"=w469) -> ("error out"=w466:errorcluster)  [unwired: 7 in]
              }
            }
            n223 = case shown="True" w407 {
              tunnel: w405 -> [_ w451]
              tunnel: w394 -> [_ w449]
              tunnel: w393 -> [_ w447]
              tunnel: w392 -> [_ w446]
              tunnel: [_ w445] -> w388
              tunnel: w387 -> [_ w444]
              frame False {
              }
              frame True {
                n224 = Build Array(w451) -> (→"Unit display D":dbl[][])
                n225 = control-ref of="Unit display D"() -> (w448:refnum<vi>)
                n226 = call "Name plot legend from array.vi"("Force write (F)"=w446, "Enabled (1-10)(1)"=w447, "Names legend"=w449, "error in (no error)"=w444, "Chart in"=w448) -> ("error out"=w445:errorcluster)  [unwired: 6 in]
              }
            }
            n227 = flat-sequence {
              tunnel: w386 -> [w420]
              tunnel: [w420] -> w385
              frame #0 {
                n228 = local write "update_legends"(FALSE ("update_legends")) -> ()
              }
            }
            n229 = Merge Errors(w391, w390, w389, w388) -> (w386:errorcluster)
          }
        }
      }
      frame True {
        # "or stop received"
        # "dequeue timed out\nno message to read"
      }
    }
    n230 = Or(x=w293, y=w292) -> (x .or. y?=w294:bool)
  }
  n231 = while {
    tunnel: w31 -> [w515]
    tunnel: w30 -> [w511]
    tunnel: [w510] -> _
    stop <- w509 stop-if-true
    # "UI process loop"
    n232 = Wait on Notification(notifier=w515, timeout in ms (-1)=-1) -> (notification=w514:T4, error out=w512:errorcluster)  [unwired: 2 in, 2 out]
    n233 = case shown="\"MEAS_TRIG_ON\"" w514 {
      tunnel: [_ _ _ _ _ TRUE _] -> w513
      tunnel: [w517 w555 w586 w607 w648 w689 w691] -> w510
      tunnel: w512 -> [w530 w564 w591 w606 w652 w689 w691]
      tunnel: w511 -> [w534 w569 w592 w608 w653 _ _]
      frame "SENS_PWR_ALL_ON_OFF" {
        # "wait for units to answer, processed in read process loop."
        # "value all used ports ON"
        # "ms"
        # "if any is 1, put all to 0,\nif all are 1, put all to 0\nif all are 0, put all to 1"
        n234 = local read "ACK'd_clients addr"() -> (w527:u32[])
        n235 = local read "Sensor power control"() -> (w532:T2)
        n236 = invoke on="Answer_received_from" class="Arr (strict)" method="Reinit To Default"(error in=w530) -> (error out=w529:errorcluster)  [unwired: 2 in, 2 out]
        n237 = call "Power_ctrl_to_ioEXPSET.vi"("error in (no error)"=w529, "Sensor power control"=w532) -> ("error out"=w521:errorcluster, "IO expaneder setting out"=w531:u16)  [unwired: 7 in, 1 out]
        n238 = flat-sequence {
          tunnel: w521 -> [_]
          tunnel: w520 -> [w536]
          tunnel: [w535] -> w519
          frame #0 {
            n239 = call "Power_ctrl_to_ioEXPSET.vi"("IO exp. setting in"=w536) -> ("error out"=w535:errorcluster, "Sensor power out"=w537:T2)  [unwired: 8 in, 1 out]
            n240 = local write "Sensor power control"(w537) -> ()
          }
        }
        n241 = case shown="Default" w531 {
          tunnel: [u16 0 ("t") u16 65472 ("t")] -> w520
          frame Default {
          }
          frame 0 {
          }
        }
        n242 = local read "ACK'd_clients"() -> (w522:u8[])
        n243 = local read "Unit port"() -> (w518:u16)
        n244 = call "Write_sensor_power.vi"("send to port (65500)"=w518, "error in (no error)"=w519, "ACK'd_clients addr"=w527, "IO expander data to write"=w520, "UDP Send Queue in"=w534) -> ("error out"=w526:errorcluster)  [unwired: 6 in]
        n245 = for {
          N: 5000 -> [_]
          tunnel: w522 -> [w547]
          tunnel: [w543] -> w523
          tunnel: w526 -> [w542]
          tunnel: [w542] -> w525
          stop <- w543 stop-if-true
          # "T - ok\nF - timed out"
          n246 = local read "Answer_received_from"() -> (w546:u8[])
          n247 = for {
            tunnel: w547 -> [w552] mode=indexing
            tunnel: w546 -> [w551]
            tunnel: [w548] -> w545
            stop <- w548 stop-if-true
            # "end\nfalse\nall found"
            n248 = Search 1D Array(1D array=w551, element=w552) -> (index of element=w550:i32)  [unwired: 1 in]
            n249 = Equal?(x=w550, y=-1) -> (x = y?=w548:bool)
          }
          n250 = Not(x=w545) -> (.not. x?=w543:bool)
          n251 = Wait (ms)(milliseconds to wait=u32 1) -> ()  [unwired: 1 out]
        }
        n252 = property on="Power all sensors ON/OFF" class="Bool"(error in=w525, "DisabledEnum"=T6."Enabled" ("Disabled")) -> (error out=w524:errorcluster)  [unwired: 1 in, 1 out]
        n253 = case shown="False" w523 {
          tunnel: w524 -> [w538 w540]
          tunnel: [w538 w540] -> w517
          frame True {
            n254 = local write "Status"("Power write OK,Ready!" ("Status")) -> ()
          }
          frame False {
            n255 = local write "Status"("Power write failed, Ready" ("Status")) -> ()
          }
        }
      }
      frame "SENS_PWR_CTRL" {
        # "ms"
        # "if any is 1, put all to 0,\nif all are 1, put all to 0\nif all are 0, put all to 1"
        n256 = local read "Sensor power control"() -> (w568:T2)
        n257 = invoke on="Answer_received_from" class="Arr (strict)" method="Reinit To Default"(error in=w564) -> (error out=w563:errorcluster)  [unwired: 2 in, 2 out]
        n258 = call "Power_ctrl_to_ioEXPSET.vi"("error in (no error)"=w563, "Sensor power control"=w568) -> ("error out"=w567:errorcluster, "IO expaneder setting out"=w565:u16)  [unwired: 7 in, 1 out]
        n259 = local read "ACK'd_clients addr"() -> (w570:u32[])
        n260 = local read "ACK'd_clients"() -> (w557:u8[])
        n261 = local read "Unit port"() -> (w556:u16)
        n262 = call "Write_sensor_power.vi"("send to port (65500)"=w556, "error in (no error)"=w567, "ACK'd_clients addr"=w570, "IO expander data to write"=w565, "UDP Send Queue in"=w569) -> ("error out"=w558:errorcluster)  [unwired: 6 in]
        n263 = for {
          N: 5000 -> [_]
          tunnel: w557 -> [w580]
          tunnel: [w576] -> w561
          tunnel: w558 -> [w575]
          tunnel: [w575] -> w559
          stop <- w576 stop-if-true
          # "T - ok\nF - timed out"
          n264 = local read "Answer_received_from"() -> (w579:u8[])
          n265 = for {
            tunnel: w580 -> [w585] mode=indexing
            tunnel: w579 -> [w584]
            tunnel: [w581] -> w578
            stop <- w581 stop-if-true
            # "end\nfalse\nall found"
            n266 = Search 1D Array(1D array=w584, element=w585) -> (index of element=w583:i32)  [unwired: 1 in]
            n267 = Equal?(x=w583, y=-1) -> (x = y?=w581:bool)
          }
          n268 = Not(x=w578) -> (.not. x?=w576:bool)
          n269 = Wait (ms)(milliseconds to wait=u32 1) -> ()  [unwired: 1 out]
        }
        n270 = case shown="False" w561 {
          tunnel: w559 -> [w571 w573]
          tunnel: [w571 w573] -> w560
          frame True {
            n271 = local write "Status"("Power write OK,Ready!" ("Status")) -> ()
          }
          frame False {
            n272 = local write "Status"("Power write failed, Ready" ("Status")) -> ()
          }
        }
        n273 = property on="Sensor power control" class="Clust (strict)"(error in=w560, "DisabledEnum"=T6."Enabled" ("Disabled")) -> (error out=w555:errorcluster)  [unwired: 1 in, 1 out]
      }
      frame "UNIT_RESET" {
        n274 = local read "Unit selection merged"() -> (w589:u8[][])
        n275 = Index Array(array=w589, index (col)=0 ("disabled index (col)")) -> (element=w587:u8[])  [unwired: 1 in]
        n276 = for {
          tunnel: w592 -> [w604]
          tunnel: w591 -> [w603]
          tunnel: [w594] -> w586
          tunnel: w587 -> [w593] mode=indexing
          stop <- w594 stop-if-true
          w596 = u8 2  # command #
          n277 = local read "Unit port"() -> (w595:u16)
          n278 = call "Send_simple_command.vi"("Unit selection"=w593, "Unit port"=w595, "cmd #"=w596) -> ("Cluster"=w597:T5)  [unwired: 8 in]
          n279 = Format Into String(format string="%d", initial string="Reset sent to #" ("string"), w593) -> (resulting string=w600:string)  [unwired: 1 in, 1 out]
          n280 = Enqueue Element(queue=w604, element=w597, timeout in ms (-1)=50, error in (no error)=w603) -> (error out=w601:errorcluster)  [unwired: 2 out]
          n281 = call "Status send Error cluster.vi"("error in (no error)"=w601, "Send status msg \"XXX\" or don't wire for no message"=w600) -> ("error out"=w594:errorcluster)  [unwired: 7 in]
        }
        n282 = local write "Status"("Reset sent, Ready!" ("Status")) -> ()
      }
      frame "MEAS_TRIG_ON" {
        n283 = local read "Unit selection merged"() -> (w605:u8[][])
        n284 = for {
          tunnel: w608 -> [w647]
          tunnel: [w620] -> w607
          tunnel: w606 -> [w632]
          tunnel: w605 -> [w619] mode=indexing
          stop <- w620 stop-if-true
          w644 = u8 3  # cmd #
          n285 = Index Array(array=w619, index=0) -> (element=w609:u8)
          n286 = Index Array(array=w619, index=1) -> (element=w610:u8)
          n287 = Index Array(array=w619, index=2) -> (element=w615:u8)
          n288 = local read "Export Folder Path"() -> (w633:path)
          n289 = Equal To 0?(x=w615) -> (x = 0?=w614:bool)
          n290 = local read "Data file ref"() -> (w623:refnum<file>)
          n291 = Select(t=u8 0, s=w614, f=u8 1) -> (s? t:f=w611:u8)
          n292 = Multiply(x=sgl 10.0, y="Period (s)") -> (x*y=w636:sgl)
          n293 = call "Create_data_log_file.vi"("error in (no error)"=w632, "Export Folder Path"=w633, "Byte Stream File in"=w623) -> ("error out"=w631:errorcluster, "Byte Stream File out"=→"Data file ref":refnum<file>)  [unwired: 7 in]
          n294 = Round Toward +Infinity(x=w636) -> (ceil(x): smallest int >= x=w635:sgl)
          n295 = To Unsigned Byte Integer(number=w635) -> (unsigned 8bit integer=w621:u8)
          n296 = Logical Shift(y=i16 1, x=w610) -> (x << y=w627:u8)
          n297 = Add(x=w627, y=w611) -> (x+y=w625:u8)
          n298 = local read "Unit port"() -> (w642:u16)
          n299 = Build Array(w621, w625, "TIACN", "REFCN", "MODECN") -> (w634:u8[])
          n300 = call "Send_simple_command.vi"("index5 array"=w634, "Unit selection"=w609, "Unit port"=w642, "cmd #"=w644) -> ("Cluster"=w646:T5)  [unwired: 7 in]
          n301 = Enqueue Element(queue=w647, element=w646, timeout in ms (-1)=50, error in (no error)=w631) -> (error out=w641:errorcluster)  [unwired: 2 out]
          n302 = local write "Status"("Trigger sent, Ready!" ("Status")) -> ()
          n303 = Format Into String(format string="%d, T=%d00ms, conf.set %d, ammonia %d", initial string="Trigger sent to #" ("string"), w609, w621, w610, w611) -> (resulting string=w640:string)  [unwired: 1 in, 1 out]
          n304 = call "Status send Error cluster.vi"("error in (no error)"=w641, "Send status msg \"XXX\" or don't wire for no message"=w640) -> ("error out"=w620:errorcluster)  [unwired: 7 in]
        }
      }
      frame "MEAS_TRIG_OFF" {
        n305 = local read "Unit selection merged"() -> (w651:u8[][])
        n306 = Index Array(array=w651, index (col)=0 ("disabled index (col)")) -> (element=w649:u8[])  [unwired: 1 in]
        n307 = for {
          N -> [w658]
          tunnel: w653 -> [w672]
          tunnel: w652 -> [w671]
          tunnel: [w659] -> w648
          tunnel: w649 -> [w654] mode=indexing
          i -> [w656]
          stop <- w659 stop-if-true
          w662 = u32 10  # milliseconds to wait (0)
          w668 = u8 4  # cmd #
          # "execute on last item in array"
          # "keep some time to receive last data before closing file"
          n308 = local read "Unit port"() -> (w667:u16)
          n309 = call "Send_simple_command.vi"("Unit selection"=w654, "Unit port"=w667, "cmd #"=w668) -> ("Cluster"=w670:T5)  [unwired: 8 in]
          n310 = Enqueue Element(queue=w672, element=w670, timeout in ms (-1)=50, error in (no error)=w671) -> (error out=w666:errorcluster)  [unwired: 2 out]
          n311 = Format Into String(format string="%d", initial string="Stop sent to #" ("string"), w654) -> (resulting string=w665:string)  [unwired: 1 in, 1 out]
          n312 = call "Status send Error cluster.vi"("error in (no error)"=w666, "milliseconds to wait (0)"=w662, "Send status msg \"XXX\" or don't wire for no message"=w665) -> ("error out"=w661:errorcluster)  [unwired: 6 in]
          n313 = flat-sequence {
            tunnel: [w687] -> _
            tunnel: w661 -> [w687]
            tunnel: [w687] -> w660
            frame #0 {
              n314 = local write "Status"("Trigger OFF sent, Ready!" ("Status")) -> ()
            }
          }
          n315 = Decrement(x=w658) -> (x-1=w657:i32)
          n316 = Equal?(x=w657, y=w656) -> (x = y?=w655:bool)
          n317 = case shown="True" w655 {
            tunnel: [w673 w677] -> w659
            tunnel: w660 -> [w673 w675]
            frame False {
              # "keep file"
            }
            frame True {
              # "close file"
              n318 = local read "Data file ref"() -> (w679:refnum<file>)
              n319 = call "Status send Error cluster.vi"("error in (no error)"=w675, "milliseconds to wait (0)"=u32 500) -> ("error out"=w676:errorcluster)  [unwired: 7 in]
              n320 = Not A Number/Path/Refnum?(number/path/refnum=w679) -> (NaN/Path/Refnum?=w678:bool)
              n321 = case shown="False" w678 {
                tunnel: w679 -> [w680 _]
                tunnel: [w681 w685] -> w677
                tunnel: w676 -> [w682 w683]
                frame False {
                  n322 = Close File(refnum=w680, error in=w682) -> (error out=w681:errorcluster)  [unwired: 1 out]
                }
                frame True {
                  n323 = local write "Status"("Error (check log), Ready!" ("Status")) -> ()
                  n324 = call "Status send Error cluster.vi"("error in (no error)"=w683, "Send status msg \"XXX\" or don't wire for no message"="ERROR: Measurement was not logged to file." ("Status")) -> ("error out"=w685:errorcluster)  [unwired: 7 in]
                }
              }
            }
          }
        }
      }
      frame "STOP" {
      }
      frame Default {
      }
    }
    n325 = Or(x=w513, y=w510) -> (x .or. y?=w509:bool)
  }
  n326 = call-poly "loop error, restart vi_polymorphic.vi"("error in (no error)"=w5) -> ()  [unwired: 11 in]
  n327 = call <vilib>:"Simple Error Handler.vi"("error in (no error)"=w5) -> ("error out"=w8:errorcluster)  [unwired: 4 in, 4 out]
  n328 = Release Notifier(notifier=w45, error in (no error)=w44) -> (error out=w42:errorcluster)  [unwired: 1 in, 2 out]
  n329 = Release Queue(queue=w34, force destroy? (F)=TRUE, error in (no error)=w42) -> (error out=w41:errorcluster)  [unwired: 2 out]
  n330 = Release Queue(queue=w30, force destroy? (F)=TRUE, error in (no error)=w41) -> (error out=w40:errorcluster)  [unwired: 2 out]
  n331 = call-poly "loop error, restart vi_polymorphic.vi"("error in (no error)"=w2) -> ()  [unwired: 11 in]
  n332 = UDP Close(connection ID=w35, 8:w40) -> (error out=w4:errorcluster)  [unwired: 1 out]
  n333 = call <vilib>:"Simple Error Handler.vi"("error in (no error)"=w2) -> ()  [unwired: 4 in, 5 out]
  n334 = call-poly "loop error, restart vi_polymorphic.vi"("error in (no error)"=w3) -> ()  [unwired: 11 in]
  n335 = call <vilib>:"Simple Error Handler.vi"("error in (no error)"=w3) -> ()  [unwired: 4 in, 5 out]
  n336 = call-poly "loop error, restart vi_polymorphic.vi"() -> ()  [unwired: 12 in]
  n337 = call <vilib>:"Simple Error Handler.vi"() -> ("error out"=w9:errorcluster)  [unwired: 5 in, 4 out]
  n338 = call-poly "loop error, restart vi_polymorphic.vi"("error in (no error)"=w4) -> ()  [unwired: 11 in]
  n339 = call <vilib>:"Simple Error Handler.vi"("error in (no error)"=w4) -> ()  [unwired: 4 in, 5 out]
  n340 = Merge Errors(w8, w4, w3, w2, w9) -> (w43:errorcluster)
  n341 = flat-sequence {
    tunnel: w43 -> [_]
    frame #0 {
      n342 = local write "Status"("Stopped" ("Status")) -> ()
    }
  }
